vi "Variables_Offset.vi"() -> ()   [LabVIEW 2015]
panel:
  out "Boolean 5":bool
  out "Boolean 4":bool
  out "Boolean 3":bool
  out "Boolean 2":bool
  out "Boolean":bool
  out "valor 5":dbl
  out "valor 4":dbl
  out "valor 3":dbl
  out "valor 2":dbl
  out "valor 1":dbl
  out "LVDTVolOff":bool
  out "PresCamaraOff":bool
  out "PresPoroOff":bool
  out "LVDTAxOff":bool
  out "CCargaOff":bool
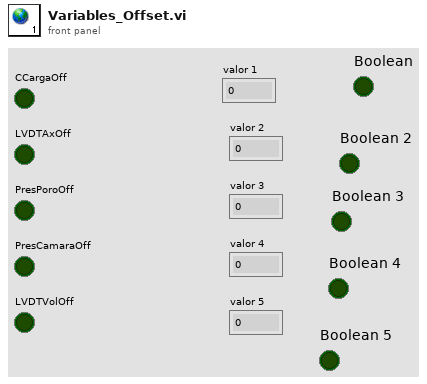
[diagram p1: front panel]
diagram:
